vi "Update Graphs.vi"(8 "error in (no error)":errorcluster, 11 "Sensor & Control in":refnum<class "Sensor & Control.lvclass">) -> (0 "error out":errorcluster, 3 "Sensor & Control out":refnum<class "Sensor & Control.lvclass">)   [LabVIEW 2013, in "Sensor & Control.lvib.lvlib" / "Sensor & Control.lvclass"]
uses:
  Sensor & Control.lvclass
  Sensor & Control.lvclass/Sensor & Control.ctl
  Read Graph History.vi
  Read Graph.vi
  Read Setpoint.vi
  PluginInterface/PluginInterface.lvlibp/PluginInterfaceClass/Read TDMS.vi
  PluginInterface/PluginInterface.lvlibp/PluginInterfaceClass/Read Name.vi
  PluginInterface/PluginInterface.lvlibp/PluginInterfaceClass/Read DVR.vi
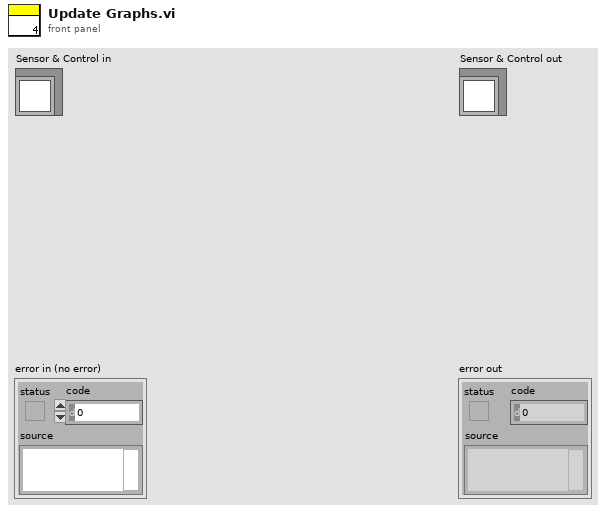
[diagram p1: front panel]
types:
  T1 = cluster{"output array":dbl[], "output array":dbl[]}
  T2 = cluster{"output array":dbl[], "output array":dbl[]}[]
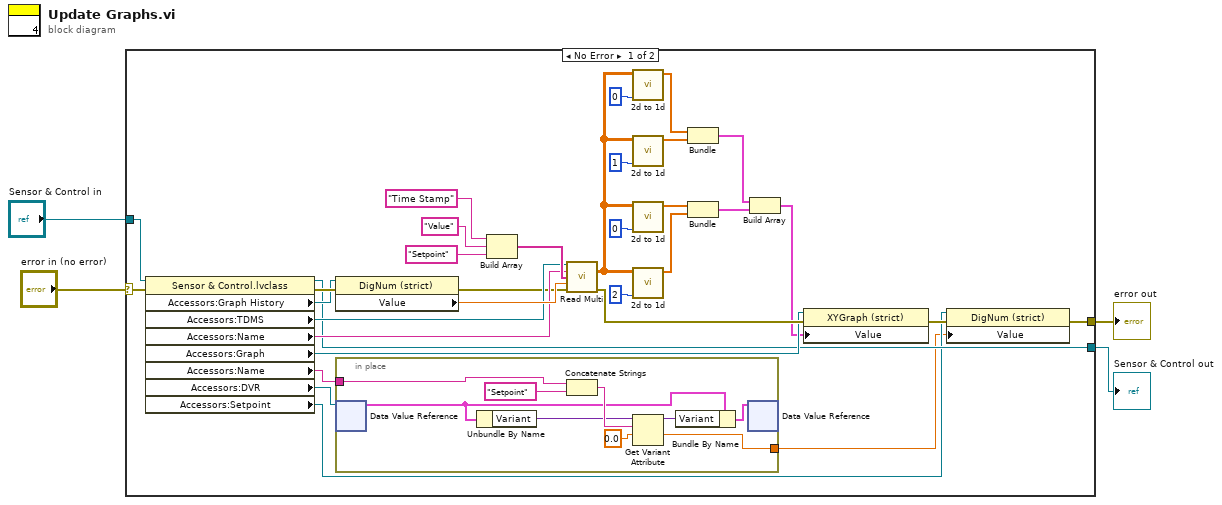
[diagram p0: block diagram]
diagram:
  n1 = case shown="No Error" "error in (no error)" {
    selector: "error in (no error)" -> [w33 w48]
    tunnel: [w9 w48] -> w1
    tunnel: [w11 w47] -> w2
    tunnel: "Sensor & Control in" -> [w37 w47]
    frame No Error {
      n2 = property class="Sensor & Control.lvclass"(reference=w37, error in=w33) -> (reference out=w11:refnum<class "Sensor & Control.lvclass">, error out=w32:errorcluster, "Accessors:Graph History"=w28:refnum<vi>, "Accessors:TDMS"=w29:refnum<k34>, "Accessors:Name"=w13:string, "Accessors:Graph"=w26:refnum<vi>, "Accessors:Name"=w6:string, "Accessors:DVR"=w7:refnum<data-value>, "Accessors:Setpoint"=w8:refnum<vi>)
      n3 = property class="DigNum (strict)"(reference=w28, error in=w32) -> (error out=w12:errorcluster, "Value"=w30:dbl)  [unwired: 1 out]
      n4 = in-place {
        in-place-border: w6 -> [w46]
        in-place-border: [w45] -> w5
        n5 = in-place-dvr #1(w7) -> (w41:cluster{"Array":string[], "Variant":variant})  [unwired: 1 out]
        n6 = Unbundle By Name(w41) -> ("Variant"=w40:variant)
        n7 = Concatenate Strings(w46, "Setpoint" ("string")) -> (w42:string)
        n8 = Get Variant Attribute(Variant=w40, name=w42, default value (empty Variant)=0.0 ("Value")) -> (duplicate Variant=w39:variant, value=w45:dbl)  [unwired: 1 in, 2 out]
        n9 = Bundle By Name(cluster=w41, "Variant"=w39) -> (w38:cluster{"Array":string[], "Variant":variant})
        n10 = in-place-dvr #1(w38) -> ()  [unwired: 2 out]
      }
      n11 = Build Array("Time Stamp" ("Channel"), "Value" ("string"), "Setpoint" ("string")) -> (w31:string[])
      n12 = call "Read Multi.vi"("tdms file in"=w29, "group"=w13, "Channel"=w31, "Numeric"=w30, "error in (no error)"=w12) -> ("Array"=w17:dbl[][], "error out"=w27:errorcluster)  [unwired: 7 in, 2 out]
      n13 = call "2d to 1d.vi"("index"=0, "array"=w17) -> ("output array"=w20:dbl[])  [unwired: 9 in]
      n14 = call "2d to 1d.vi"("index"=1, "array"=w17) -> ("output array"=w15:dbl[])  [unwired: 9 in]
      n15 = call "2d to 1d.vi"("index"=0, "array"=w17) -> ("output array"=w21:dbl[])  [unwired: 9 in]
      n16 = call "2d to 1d.vi"("index"=2, "array"=w17) -> ("output array"=w14:dbl[])  [unwired: 9 in]
      n17 = Bundle("output array"=w20, "output array"=w15) -> (w19:T1)  [unwired: 1 in]
      n18 = Bundle("output array"=w21, "output array"=w14) -> (w18:T1)  [unwired: 1 in]
      n19 = Build Array(w19, w18) -> (w16:T2)
      n20 = property class="XYGraph (strict)"(reference=w26, error in=w27, "Value"=w16) -> (error out=w10:errorcluster)  [unwired: 1 out]
      n21 = property class="DigNum (strict)"(reference=w8, error in=w10, "Value"=w5) -> (error out=w9:errorcluster)  [unwired: 1 out]
    }
    frame Error {
    }
  }
  "error out" <- w1
  "Sensor & Control out" <- w2
